vi "UTF8String to BGI encoding string.vi"(11 "Line1":string) -> (3 "String":string)   [LabVIEW 2019]
doc: "This VI is Developed by Anish Prabu T.\n\nCopyright © 2006, email:anishprabu243@yahoo.co.in.\nAll rights reserved."
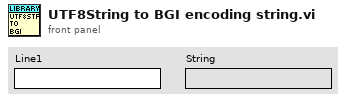
[diagram p1: front panel]
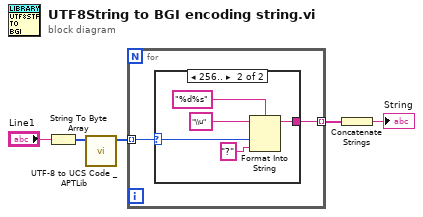
[diagram p0: block diagram]
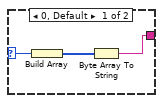
[diagram p2: hidden frame]
diagram:
  n1 = String To Byte Array(string="Line1") -> (unsigned byte array=w2:u8[])
  n2 = call <userlib>:"UTF-8 to UCS Code _APTLib.vi"("[UTF-8]"=w2) -> ("[UCS]"=w3:u32[])  [unwired: 8 in, 2 out]
  n3 = for {
    tunnel: w3 -> [w6] mode=indexing
    tunnel: [w7] -> w4 mode=indexing
    n4 = case shown="256.." w6 {
      selector: w6 -> [w10 w11]
      tunnel: [w9 w12] -> w7
      frame 0, Default {
        n5 = Build Array(w10) -> (w8:u32[])
        n6 = Byte Array To String(unsigned byte array=w8) -> (string=w9:string)
      }
      frame 256.. {
        n7 = Format Into String(format string="%d%s", initial string="\\u", w11, "?" ("initial string")) -> (resulting string=w12:string)  [unwired: 1 in, 1 out]
      }
    }
  }
  n8 = Concatenate Strings(w4) -> (→"String":string)
